vi "addToResultsQ.vi"(8 "error in (no error)":errorcluster, 10 "Results":string, 11 "AnalysisFile in":refnum<class "AnalysisFile.lvclass">) -> (0 "error out":errorcluster, 3 "AnalysisFile out":refnum<class "AnalysisFile.lvclass">)   [LabVIEW 2009, in "Views.lvlib" / "Camera.lvlib" / "AnalysisFile.lvclass"]
uses:
  AnalysisFile.lvclass
  Tools/Filing/FileNeologist/FileNeologist.lvclass
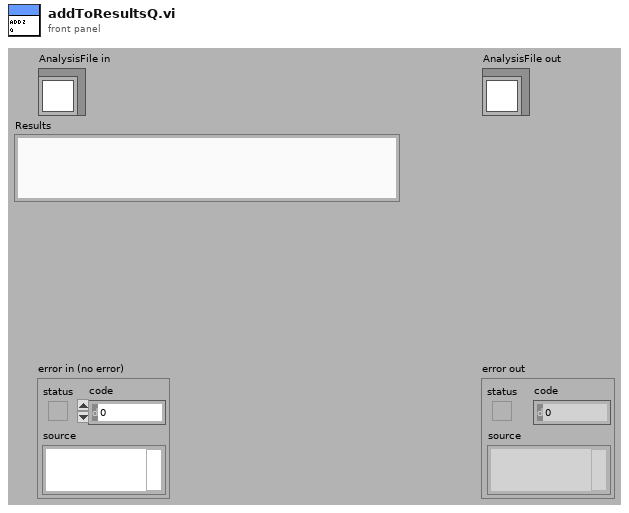
[diagram p1: front panel]
types:
  T1 = cluster{"Name":string, "Results":dbl[], "AnalysisType":string}
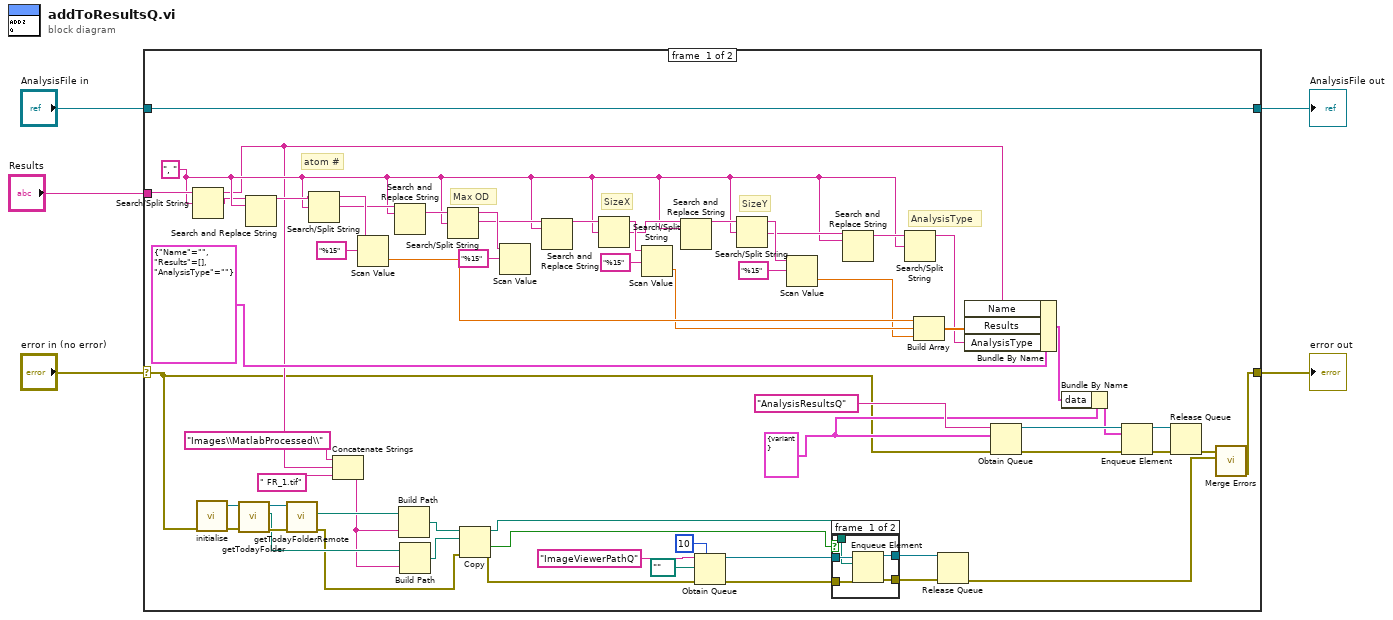
[diagram p0: block diagram]
diagram:
  n1 = case shown="No Error" "error in (no error)" {
    selector: "error in (no error)" -> [w22 w76]
    tunnel: [w19 w76] -> w4
    tunnel: [w67 w75] -> w2
    tunnel: "AnalysisFile in" -> [w67 w75]
    tunnel: "Results" -> [w66 _]
    frame #0 {
      w36 = cluster{"data":variant} {"data"=variant} ("dataQ")
      w42 = ", "
      # "AnalysisType"
      # "SizeY"
      # "SizeX"
      # "Max OD"
      # "atom #"
      n2 = Search/Split String(string=w66, search string/char (-)=w42) -> (substring before match=w28:string, match + rest of string=w33:string)  [unwired: 1 in, 1 out]
      n3 = call "initialise.vi"("error in (no error)"=w22) -> ("error out"=w29:errorcluster, "FileNeologist out"=w30:refnum<class "FileNeologist.lvclass">)  [unwired: 9 in]
      n4 = call "getTodayFolder.vi"("error in (no error)"=w29, "FileNeologist in"=w30) -> ("error out"=w31:errorcluster, "todayFolder"=w25:path, "FileNeologist out"=w32:refnum<class "FileNeologist.lvclass">)  [unwired: 7 in]
      n5 = Search and Replace String(input string=w33, search string=w42) -> (result string=w53:string)  [unwired: 6 in, 3 out]
      n6 = call "getTodayFolderRemote.vi"("error in (no error)"=w31, "FileNeologist in"=w32) -> ("error out"=w23:errorcluster, "todayFolder"=w26:path)  [unwired: 7 in, 1 out]
      n7 = Search/Split String(string=w53, search string/char (-)=w42) -> (substring before match=w65:string, match + rest of string=w52:string)  [unwired: 1 in, 1 out]
      n8 = Concatenate Strings("Images\\MatlabProcessed\\", w28, " FR_1.tif") -> (w24:string)
      n9 = Scan Value(string=w65, format string="%15") -> (value=w58:dbl)  [unwired: 1 in, 1 out]
      n10 = Search and Replace String(input string=w52, search string=w42) -> (result string=w51:string)  [unwired: 6 in, 3 out]
      n11 = Build Path(base path=w26, name or relative path=w24) -> (appended path=w17:path)
      n12 = Build Path(base path=w25, name or relative path=w24) -> (appended path=w16:path)
      n13 = Search/Split String(string=w51, search string/char (-)=w42) -> (substring before match=w61:string, match + rest of string=w49:string)  [unwired: 1 in, 1 out]
      n14 = Copy(8:w23, 10:w16, 11:w17) -> (0:w6:errorcluster, 1:w8:bool, 3:w7:path)  [unwired: 2 in]
      n15 = Scan Value(string=w61, format string="%15") -> ()  [unwired: 1 in, 2 out]
      n16 = Search and Replace String(input string=w49, search string=w42) -> (result string=w50:string)  [unwired: 6 in, 3 out]
      n17 = Search/Split String(string=w50, search string/char (-)=w42) -> (substring before match=w47:string, match + rest of string=w46:string)  [unwired: 1 in, 1 out]
      n18 = Scan Value(string=w47, format string="%15") -> (value=w57:dbl)  [unwired: 1 in, 1 out]
      n19 = Search and Replace String(input string=w46, search string=w42) -> (result string=w48:string)  [unwired: 6 in, 3 out]
      n20 = Obtain Queue(max queue size (-1, unlimited)=10, name (unnamed)="ImageViewerPathQ", element data type=path "", error in (no error)=w6) -> (queue out=w12:refnum<queue>, error out=w11:errorcluster)  [unwired: 1 in, 1 out]
      n21 = Search/Split String(string=w48, search string/char (-)=w42) -> (substring before match=w45:string, match + rest of string=w43:string)  [unwired: 1 in, 1 out]
      n22 = Scan Value(string=w45, format string="%15") -> (value=w56:dbl)  [unwired: 1 in, 1 out]
      n23 = case shown="False" w8 {
        tunnel: w12 -> [w72 w74]
        tunnel: w11 -> [w71 w73]
        tunnel: w7 -> [w70 _]
        tunnel: [w69 w74] -> w10
        tunnel: [w68 w73] -> w9
        frame #0 {
          n24 = Enqueue Element(queue=w72, element=w70, error in (no error)=w71) -> (queue out=w69:refnum<queue>, error out=w68:errorcluster)  [unwired: 1 in, 1 out]
        }
        frame #1 {
        }
      }
      n25 = Search and Replace String(input string=w43, search string=w42) -> (result string=w44:string)  [unwired: 6 in, 3 out]
      n26 = Search/Split String(string=w44, search string/char (-)=w42) -> (substring before match=w54:string)  [unwired: 1 in, 2 out]
      n27 = Build Array(w58, w57, w56) -> (w55:dbl[])
      n28 = Release Queue(queue=w10, error in (no error)=w9) -> (error out=w20:errorcluster)  [unwired: 1 in, 2 out]
      n29 = Bundle By Name(cluster=T1 {"Name"="", "Results"=[], "AnalysisType"=""} ("output cluster"), "Name"=w28, "Results"=w55, "AnalysisType"=w54) -> (w35:T1)
      n30 = Obtain Queue(name (unnamed)="AnalysisResultsQ", element data type=w36, error in (no error)=w22) -> (queue out=w41:refnum<queue>, error out=w38:errorcluster)  [unwired: 2 in, 1 out]
      n31 = Bundle By Name(cluster=w36, "data"=w35) -> (w34:cluster{"data":variant})
      n32 = Enqueue Element(queue=w41, element=w34, error in (no error)=w38) -> (queue out=w40:refnum<queue>, error out=w39:errorcluster)  [unwired: 1 in, 1 out]
      n33 = Release Queue(queue=w40, error in (no error)=w39) -> (error out=w21:errorcluster)  [unwired: 1 in, 2 out]
      n34 = call <vilib>:"Merge Errors.vi"("error in 2 (no error)"=w20, "error in 1 (no error)"=w21) -> ("error out"=w19:errorcluster)  [unwired: 5 in]
    }
    frame #1 {
    }
  }
  "error out" <- w4
  "AnalysisFile out" <- w2
